vi "Correlation Test.vi"(6 "alternative hypothesis":i32(ring) items=["r != 0"=0, "r > 0"=1, "r < 0"=-1], 8 "significance level":dbl=0.05 format="%.4g", 9 "type":enum32{"Pearson", "Spearman", "Kendall"}(ring), 10 "sample set y":dbl[](array[numeric]), 11 "sample set x":dbl[](array[numeric])) -> (0 "error":i32, 1 "rsig":dbl, 2 "p value":dbl=0.05 format="%.6g", 3 "reject null hypothesis":bool, 4 "correlation coefficient r":dbl)   [LabVIEW 2018, in "NI_Gmath.lvlib"]
doc: "Tests hypotheses about the association between two variables x and y."
uses:
  NI_Gmath.lvlib
panel:
  # "Correlation Test\nPearson, Spearman, Kendall"
  # ">="
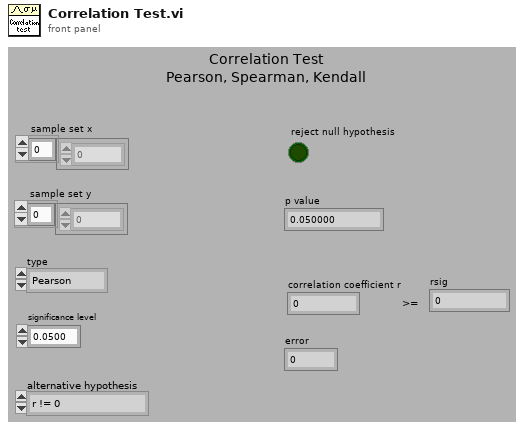
[diagram p1: front panel]
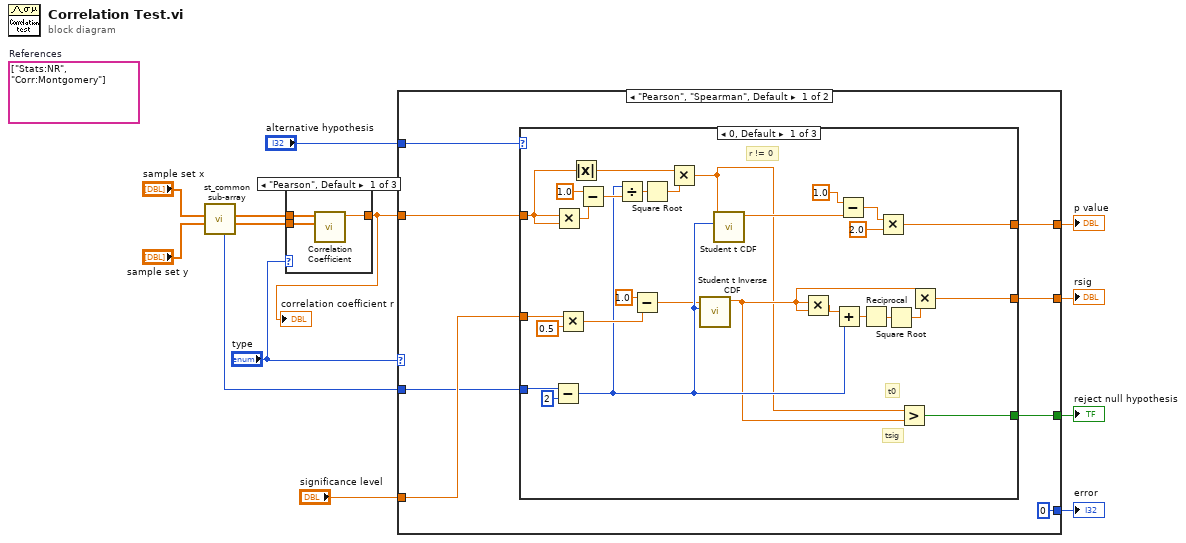
[diagram p0: block diagram]
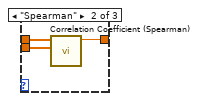
[diagram p2: hidden frame]
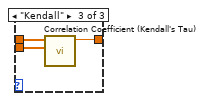
[diagram p3: hidden frame]
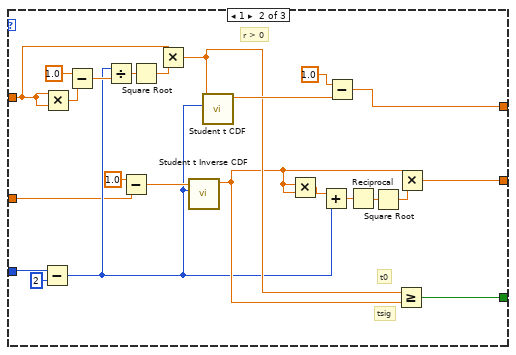
[diagram p4: hidden frame]
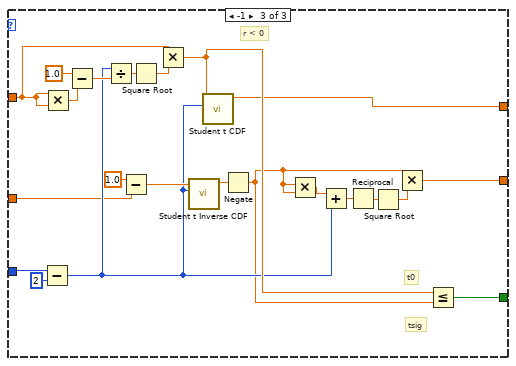
[diagram p5: hidden frame]
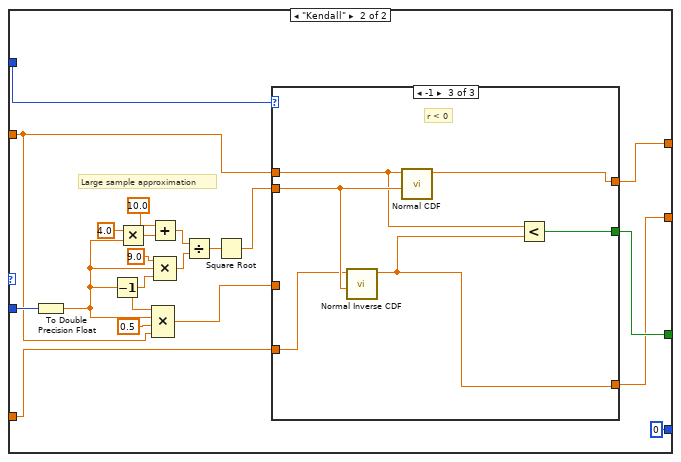
[diagram p6: hidden frame]
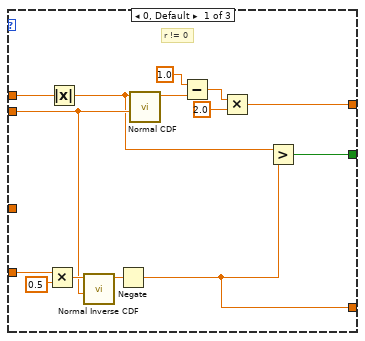
[diagram p7: hidden frame]
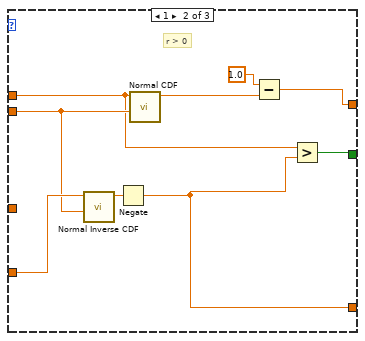
[diagram p8: hidden frame]
diagram:
  (unwired) string[] ["Stats:NR", "Corr:Montgomery"]  # References
  n1 = call "st_common sub-array.vi"(9:"array 1 in"="sample set y", 10:"array 1 in"="sample set x") -> (1:"array 1 out"=w11:dbl[], 2:"array 1 out"=w12:dbl[], "size"=w10:i32)  [unwired: 7 in]
  n2 = case shown="\"Pearson\", Default" "type" {
    tunnel: w12 -> [w16 w19 w22]
    tunnel: w11 -> [w15 w18 w21]
    tunnel: [w14 w17 w20] -> w9
    frame "Pearson", Default {
      n3 = call "Correlation Coefficient.vi"("Y"=w15, "X"=w16) -> ("correlation coefficient r"=w14:dbl)  [unwired: 8 in, 1 out]
    }
    frame "Spearman" {
      n4 = call "Correlation Coefficient (Spearman).vi"("Y"=w18, "X"=w19) -> ("correlation coefficient r"=w17:dbl)  [unwired: 8 in, 1 out]
    }
    frame "Kendall" {
      n5 = call "Correlation Coefficient (Kendall's Tau).vi"("Y"=w21, "X"=w22) -> ("correlation coefficient r"=w20:dbl)  [unwired: 8 in, 1 out]
    }
  }
  "correlation coefficient r" <- w9
  n6 = case shown="\"Pearson\", \"Spearman\", Default" "type" {
    tunnel: "significance level" -> [w30 w117]
    tunnel: w10 -> [w29 w112]
    tunnel: w9 -> [w28 w108]
    tunnel: [w27 w115] -> w8
    tunnel: [w26 w114] -> w6
    tunnel: "alternative hypothesis" -> [w25 w116]
    tunnel: [w24 w106] -> w2
    tunnel: [0 0] -> w1
    frame "Pearson", "Spearman", Default {
      n7 = case shown="0, Default" w25 {
        tunnel: w30 -> [w35 w60 w85]
        tunnel: w29 -> [w51 w78 w102]
        tunnel: [w43 w71 w95] -> w27
        tunnel: w28 -> [w32 w59 w84]
        tunnel: [w53 w61 w82] -> w26
        tunnel: [w36 w64 w88] -> w24
        frame 0, Default {
          # "tsig"
          # "t0"
          # "r != 0"
          n8 = Subtract(x=w51, y=2 ("x")) -> (x-y=w41:i32)
          n9 = Multiply(x=w32, y=w32) -> (x*y=w49:dbl)
          n10 = Multiply(x=w35, y=0.5) -> (x*y=w44:dbl)
          n11 = Absolute Value(x=w32) -> (abs(x)=w31:dbl)
          n12 = Subtract(x=1.0, y=w49) -> (x-y=w48:dbl)
          n13 = Divide(x=w41, y=w48) -> (x/y=w47:dbl)
          n14 = Subtract(x=1.0, y=w44) -> (x-y=w34:dbl)
          n15 = Square Root(x=w47) -> (sqrt(x)=w46:dbl)
          n16 = Multiply(x=w31, y=w46) -> (x*y=w33:dbl)
          n17 = call "Student t Inverse CDF.vi"("k degrees of freedom"=w41, "cdf(x)"=w34) -> ("x"=w38:dbl)  [unwired: 8 in, 1 out]
          n18 = call "Student t CDF.vi"("k degrees of freedom"=w41, "x"=w33) -> ("cdf(x)"=w56:dbl)  [unwired: 7 in, 2 out]
          n19 = Multiply(x=w38, y=w38) -> (x*y=w42:dbl)
          n20 = Add(x=w42, y=w41) -> (x+y=w40:dbl)
          n21 = Subtract(x=1.0, y=w56) -> (x-y=w54:dbl)
          n22 = Reciprocal(x=w40) -> (1/x=w39:dbl)
          n23 = Multiply(x=w54, y=2.0) -> (x*y=w53:dbl)
          n24 = Square Root(x=w39) -> (sqrt(x)=w37:dbl)
          n25 = Greater?(x=w33, y=w38) -> (0:w43:bool)
          n26 = Multiply(x=w38, y=w37) -> (x*y=w36:dbl)
        }
        frame 1 {
          # "tsig"
          # "t0"
          # "r > 0"
          n27 = Subtract(x=w78, y=2 ("x")) -> (x-y=w62:i32)
          n28 = Multiply(x=w59, y=w59) -> (x*y=w76:dbl)
          n29 = Subtract(x=1.0, y=w76) -> (x-y=w75:dbl)
          n30 = Divide(x=w62, y=w75) -> (x/y=w74:dbl)
          n31 = Subtract(x=1.0, y=w60) -> (x-y=w70:dbl)
          n32 = Square Root(x=w74) -> (sqrt(x)=w73:dbl)
          n33 = Multiply(x=w59, y=w73) -> (x*y=w69:dbl)
          n34 = call "Student t Inverse CDF.vi"("k degrees of freedom"=w62, "cdf(x)"=w70) -> ("x"=w63:dbl)  [unwired: 8 in, 1 out]
          n35 = call "Student t CDF.vi"("k degrees of freedom"=w62, "x"=w69) -> ("cdf(x)"=w80:dbl)  [unwired: 7 in, 2 out]
          n36 = Multiply(x=w63, y=w63) -> (x*y=w68:dbl)
          n37 = Add(x=w68, y=w62) -> (x+y=w67:dbl)
          n38 = Subtract(x=1.0, y=w80) -> (x-y=w61:dbl)
          n39 = Reciprocal(x=w67) -> (1/x=w66:dbl)
          n40 = Square Root(x=w66) -> (sqrt(x)=w65:dbl)
          n41 = Greater Or Equal?(x=w69, y=w63) -> (x >= y?=w71:bool)
          n42 = Multiply(x=w63, y=w65) -> (x*y=w64:dbl)
        }
        frame -1 {
          # "tsig"
          # "t0"
          # "r < 0"
          n43 = Subtract(x=w102, y=2 ("x")) -> (x-y=w86:i32)
          n44 = Multiply(x=w84, y=w84) -> (x*y=w100:dbl)
          n45 = Subtract(x=1.0, y=w100) -> (x-y=w99:dbl)
          n46 = Divide(x=w86, y=w99) -> (x/y=w98:dbl)
          n47 = Subtract(x=1.0, y=w85) -> (x-y=w94:dbl)
          n48 = Square Root(x=w98) -> (sqrt(x)=w97:dbl)
          n49 = Multiply(x=w84, y=w97) -> (x*y=w93:dbl)
          n50 = call "Student t Inverse CDF.vi"("k degrees of freedom"=w86, "cdf(x)"=w94) -> ("x"=w87:dbl)  [unwired: 8 in, 1 out]
          n51 = call "Student t CDF.vi"("k degrees of freedom"=w86, "x"=w93) -> ("cdf(x)"=w82:dbl)  [unwired: 7 in, 2 out]
          n52 = Negate(x=w87) -> (-x=w83:dbl)
          n53 = Multiply(x=w83, y=w83) -> (x*y=w92:dbl)
          n54 = Add(x=w92, y=w86) -> (x+y=w91:dbl)
          n55 = Reciprocal(x=w91) -> (1/x=w90:dbl)
          n56 = Square Root(x=w90) -> (sqrt(x)=w89:dbl)
          n57 = Multiply(x=w83, y=w89) -> (x*y=w88:dbl)
          n58 = Less Or Equal?(x=w93, y=w83) -> (x <= y?=w95:bool)
        }
      }
    }
    frame "Kendall" {
      # "Large sample approximation"
      n59 = To Double Precision Float(number=w112) -> (double precision float=w110:dbl)
      n60 = Decrement(x=w110) -> (x-1=w111:dbl)
      n61 = Multiply(x=4.0, y=w110) -> (x*y=w122:dbl)
      n62 = Add(x=10.0, y=w122) -> (x+y=w119:dbl)
      n63 = Compound Arithmetic op=MULTIPLY(w111, w110, 0.5 ("x"), w108) -> (w107:dbl)
      n64 = Compound Arithmetic op=MULTIPLY(9.0 ("x"), w110, w111) -> (w118:dbl)
      n65 = Divide(x=w119, y=w118) -> (x/y=w113:dbl)
      n66 = Square Root(x=w113) -> (sqrt(x)=w105:dbl)
      n67 = case shown="-1" w116 {
        tunnel: w117 -> [w136 w144 w149]
        tunnel: w108 -> [w133 w138 w150]
        tunnel: [w128 w142 w152] -> w114
        tunnel: [w125 w139 w148] -> w106
        tunnel: [w127 w141 w147] -> w115
        tunnel: w105 -> [w126 w140 w151]
        tunnel: w107 -> [_ _ _]
        frame 0, Default {
          # "r != 0"
          n68 = Multiply(x=w136, y=0.5) -> (x*y=w134:dbl)
          n69 = Absolute Value(x=w133) -> (abs(x)=w124:dbl)
          n70 = call "Normal Inverse CDF.vi"("std"=w126, "cdf(x)"=w134) -> ("x"=w135:dbl)  [unwired: 8 in, 1 out]
          n71 = Negate(x=w135) -> (-x=w125:dbl)
          n72 = call "Normal CDF.vi"("std"=w126, "x"=w124) -> ("cdf(x)"=w131:dbl)  [unwired: 8 in, 1 out]
          n73 = Subtract(x=1.0, y=w131) -> (x-y=w129:dbl)
          n74 = Multiply(x=w129, y=2.0) -> (x*y=w128:dbl)
          n75 = Greater?(x=w124, y=w125) -> (0:w127:bool)
        }
        frame 1 {
          # "r > 0"
          n76 = call "Normal Inverse CDF.vi"("std"=w140, "cdf(x)"=w144) -> ("x"=w143:dbl)  [unwired: 8 in, 1 out]
          n77 = Negate(x=w143) -> (-x=w139:dbl)
          n78 = call "Normal CDF.vi"("std"=w140, "x"=w138) -> ("cdf(x)"=w145:dbl)  [unwired: 8 in, 1 out]
          n79 = Subtract(x=1.0, y=w145) -> (x-y=w142:dbl)
          n80 = Greater?(x=w138, y=w139) -> (0:w141:bool)
        }
        frame -1 {
          # "r < 0"
          n81 = call "Normal Inverse CDF.vi"("std"=w151, "cdf(x)"=w149) -> ("x"=w148:dbl)  [unwired: 8 in, 1 out]
          n82 = call "Normal CDF.vi"("std"=w151, "x"=w150) -> ("cdf(x)"=w152:dbl)  [unwired: 8 in, 1 out]
          n83 = Less?(x=w150, y=w148) -> (x < y?=w147:bool)
        }
      }
    }
  }
  "error" <- w1
  "reject null hypothesis" <- w8
  "p value" <- w6
  "rsig" <- w2
